vi "CDMA_scramblingCode.vi"(6 "scramblingCode":cdb[](array[numeric]), 8 "error in (no error)":errorcluster caption="错误输入（无错误）", 10 "inputdata":cdb[](array[numeric]), 11 "Path In":path) -> (0 "error out":errorcluster caption="错误输出", 2 "outdata":cdb[](array[numeric]), 3 "Path Out":path)   [LabVIEW 2015]
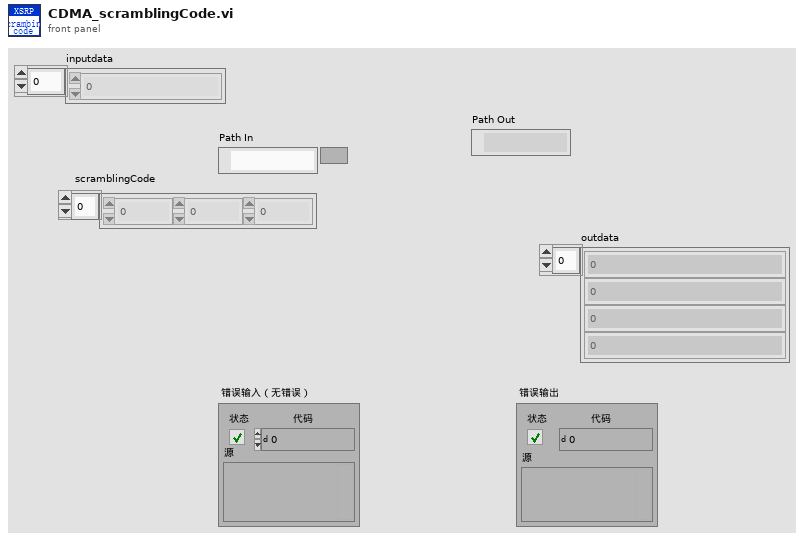
[diagram p1: front panel]
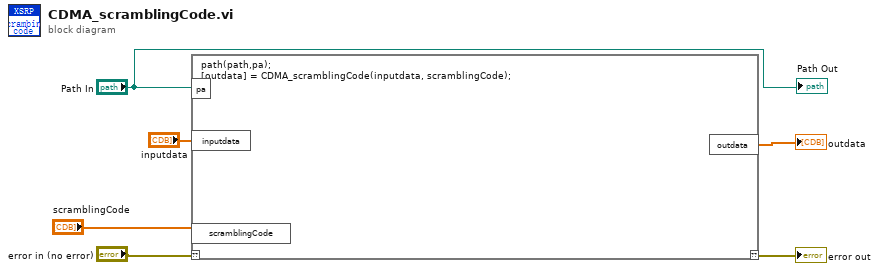
[diagram p0: block diagram]
diagram:
  n1 = script code="path(path,pa);\n[outdata] = CDMA_scramblingCode(inputdata, scramblingCode);"("??"="error in (no error)", "pa"="Path In", "scramblingCode"="scramblingCode", "inputdata"="inputdata") -> ("??"=→"error out":errorcluster, "outdata"=→"outdata":cdb[])
  "Path Out" <- "Path In"
